vi "Rotate.vi"(8 "Acceptable Error (Degrees)":dbl=0.3, 9 "Max Rotation Speed":dbl=0.4, 10 "Heading Change (Degrees)":dbl, 11 "RobotDriveDevRef":T2={"DevStatus"={"status"=FALSE, "code"=0, "source"=""}, "Motors[]"=[], "Square Inputs"=FALSE, "Max Output"=1.0, "Isochronous"=FALSE}) -> (0 "Actual Heading (Degrees)":dbl(knob)=0.4937889940289276 scale=-180.0..180.0, 3 "RobotDriveDevRef":T2={"DevStatus"={"status"=FALSE, "code"=0, "source"=""}, "Motors[]"=[], "Square Inputs"=FALSE, "Max Output"=1.0, "Isochronous"=FALSE})   [LabVIEW 2011]
uses:
  <vilib>/Rock Robotics/WPI/RobotDrive/WPI_RobotDriveDevRef.ctl
  <vilib>/Rock Robotics/WPI/MotorControl/WPI_MotorControlDeviceRef.ctl
  <vilib>/Rock Robotics/SystemInterfaces/Typedef/FPGA_TypedefDigitalModule.ctl
  <vilib>/Rock Robotics/SystemInterfaces/DIO/FPGA_DIOPWMChannel.ctl
  <vilib>/Rock Robotics/WPI/PWM/WPI_PWMDeadband.ctl
  <vilib>/Rock Robotics/WPI/CAN/Jaguar/SubVIs/WPI_CANJaguar_ControlMode.ctl
  <vilib>/Rock Robotics/WPI/PWM/WPI_PWMTransform_ConPane.ctl
  Robot Global Data.vi
  <vilib>/addons/control/pid/pid.llb/PID (DBL).vi
  <vilib>/addons/control/pid/NI_PID_pid.lvlib
panel:
  out "Rotation":dbl
  in  "StraightPID gains":T1={"proportional gain (Kc)"=0.025, "integral time (Ti, min)"=0.0, "derivative time (Td, min)"=0.0} {"derivative time (Td, min)" format="%.3f"; "integral time (Ti, min)" format="%.3f"; "proportional gain (Kc)" format="%.3f"}
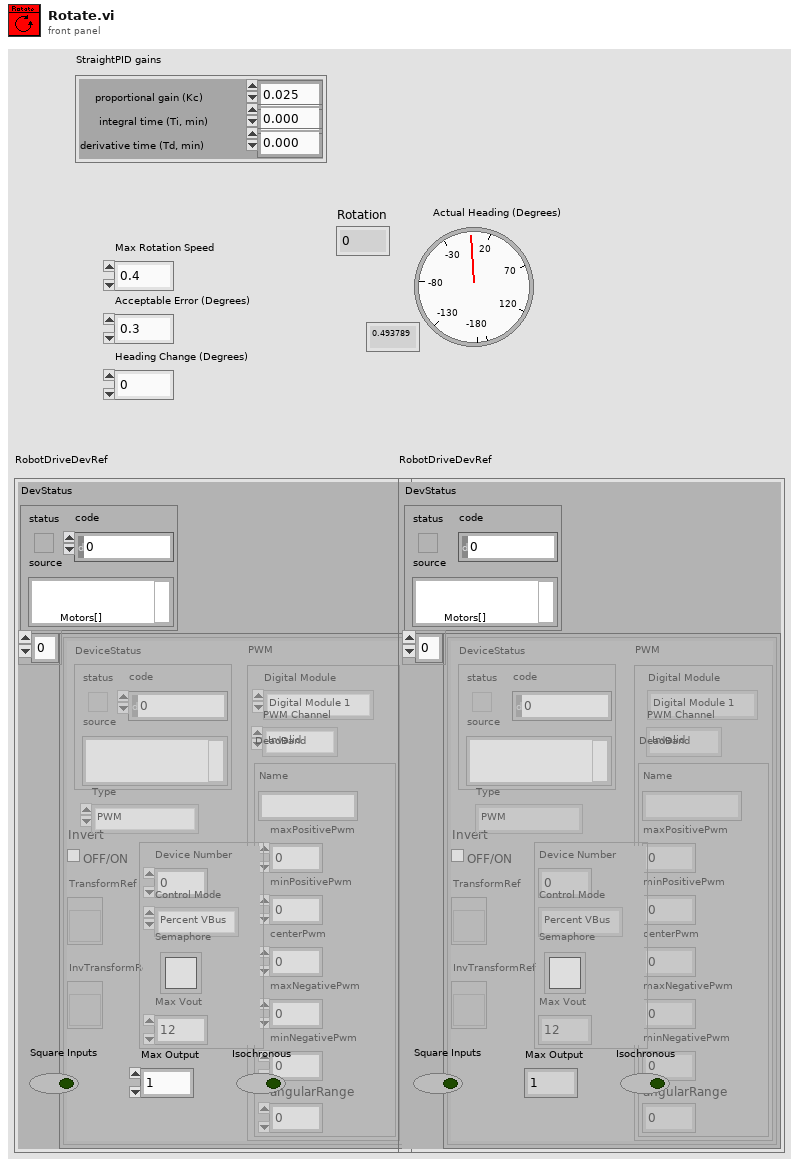
[diagram p1: front panel]
types:
  T1 = cluster{"proportional gain (Kc)":dbl, "integral time (Ti, min)":dbl, "derivative time (Td, min)":dbl}
  T2 = typedef "WPI_RobotDriveDevRef.ctl" = cluster{"DevStatus":errorcluster, "Motors[]":T3[], "Square Inputs":bool, "Max Output":dbl, "Isochronous":bool}
  T3 = typedef "WPI_MotorControlDeviceRef.ctl" = cluster{"DeviceStatus":errorcluster, "Type":enum16{"PWM", "CAN"}, "PWM":cluster{"Digital Module":T4, "PWM Channel":T5, "DeadBand":T6}, "CAN":cluster{"Device Number":u8, "Control Mode":T7, "Semaphore":T8, "Max Vout":dbl}, "Invert":bool, "TransformRef":T9, "InvTransformRef":T9}
  T4 = typedef "FPGA_TypedefDigitalModule.ctl" = enum16{"Digital Module 1", "Digital Module 2"}
  T5 = typedef "FPGA_DIOPWMChannel.ctl" = enum8{"PWM 1", "PWM 2", "PWM 3", "PWM 4", "PWM 5", "PWM 6", "PWM 7", "PWM 8", "PWM 9", "PWM 10", "Invalid"}
  T6 = typedef "WPI_PWMDeadband.ctl" = cluster{"Name":string, "maxPositivePwm":i32, "minPositivePwm":i32, "centerPwm":i32, "maxNegativePwm":i32, "minNegativePwm":i32, "angularRange":u16}
  T7 = typedef "WPI_CANJaguar_ControlMode.ctl" = enum8{"Percent VBus", "Current", "Speed", "Position", "Voltage"}
  T8 = typedef "Semaphore RefNum" = refnum<k1>
  T9 = typedef "WPI_PWMTransform_ConPane.ctl" = refnum<vi>
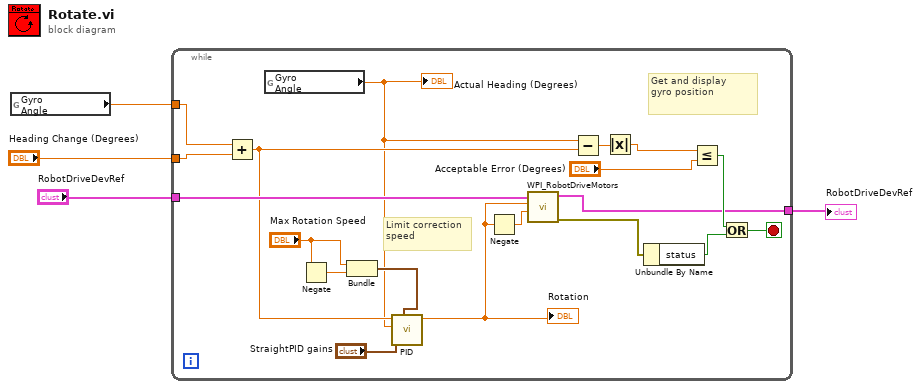
[diagram p0: block diagram]
diagram:
  n1 = global read "Robot Global Data.vi" "Gyro\nAngle"() -> (w1:dbl)
  n2 = while {
    tunnel: "RobotDriveDevRef" -> [w23]
    tunnel: "Heading Change (Degrees)" -> [w9]
    tunnel: [w11] -> w2
    tunnel: w1 -> [w10]
    stop <- w22 stop-if-true
    # "Limit correction\nspeed"
    # "Get and display\ngyro position"
    n3 = Add(x=w10, y=w9) -> (x+y=w7:dbl)
    n4 = global read "Robot Global Data.vi" "Gyro\nAngle"() -> (w5:dbl)
    "Actual Heading (Degrees)" <- w5
    n5 = Negate(x="Max Rotation Speed") -> (-x=w18:dbl)
    n6 = Bundle("Max Rotation Speed"="Max Rotation Speed", w18) -> (w17:cluster{"Max Rotation Speed":dbl, dbl})  [unwired: 1 in]
    n7 = call-poly <vilib>:"PID.vi"("output range"=w17, "PID gains"="StraightPID gains", "process variable"=w5, "setpoint"=w7) -> ("output"=w6:dbl)  [unwired: 2 in, 5 out]
    "Rotation" <- w6
    n8 = Negate(x=w6) -> (-x=w8:dbl)
    n9 = call <vilib>:"WPI_RobotDriveMotors.vi"("RightSpeed"=w8, "LeftSpeed"=w6, "RobotDriveDevRef"=w23) -> ("error out"=w21:errorcluster, "RobotDriveDevRef"=w11:T2)  [unwired: 7 in]
    n10 = Subtract(x=w5, y=w7) -> (x-y=w16:dbl)
    n11 = Absolute Value(x=w16) -> (abs(x)=w15:dbl)
    n12 = Unbundle By Name(w21) -> ("status"=w13:bool)
    n13 = Less Or Equal?(x=w15, y="Acceptable Error (Degrees)") -> (x <= y?=w12:bool)
    n14 = Or(x=w12, y=w13) -> (x .or. y?=w22:bool)
  }
  "RobotDriveDevRef" <- w2
